vi "sv_Calculate Time and Angle Positions.vi"(0 "waveform in":waveform(dbl), 2 "reset?":bool, 5 "chirp settings":T1={"amplitude"=0.0, "frequency range"={"start (Hz)"=20.0, "stop (Hz)"=20000.0, "frequency spacing"=enum."Logarithmic"}, "sampling info"={"Fs"=50000.0, "chirp duration [s]"=3.0}, "initial states"={"frequency [Hz]"=20.0, "phase [rad]"=0.0, "elapsed time [s]"=0.0}, "frequency slope"=0.0, "maximum harmonic"=0, "prefix len [samples]"={"integer"=0, "fractional"=0.0}} {"frequency slope" format="%.2f"; "prefix len [samples]"."fractional" format="%.2p"; "initial states"."elapsed time [s]" format="%.2f"; "initial states"."phase [rad]" format="%.2f"; "initial states"."frequency [Hz]" format="%.2f"; "sampling info"."chirp duration [s]" format="%.2f"; "sampling info"."Fs" format="%.2p"; "frequency range"."stop (Hz)" format="%.2f"; "frequency range"."start (Hz)" format="%.2f"; "amplitude" format="%.2f"}, 11 "error in (no error)":errorcluster) -> (4 "waveform out":waveform(dbl), 6 "time array [s]":dbl[](array[numeric]), 8 "phase array [rad]":dbl[](array[numeric]), 10 "samples/rev":i32, 15 "error out":errorcluster)   [LabVIEW 2017, in "SoundVib_ContSweptSine.lvlib"]
uses:
  <vilib>/addons/Sound and Vibration/svt_Continuous Swept Sine/SoundVib_ContSweptSine.lvlib
  <vilib>/addons/_NISVFA/_Generation/subVIs/sv_Chirp Settings.ctl
  <vilib>/addons/Sound and Vibration/svt_Continuous Swept Sine/subVIs/sv_Continuous Swept-Sine Errors.ctl
  <vilib>/addons/_NISVFA/_Generation/SoundVib_Generation.lvlib
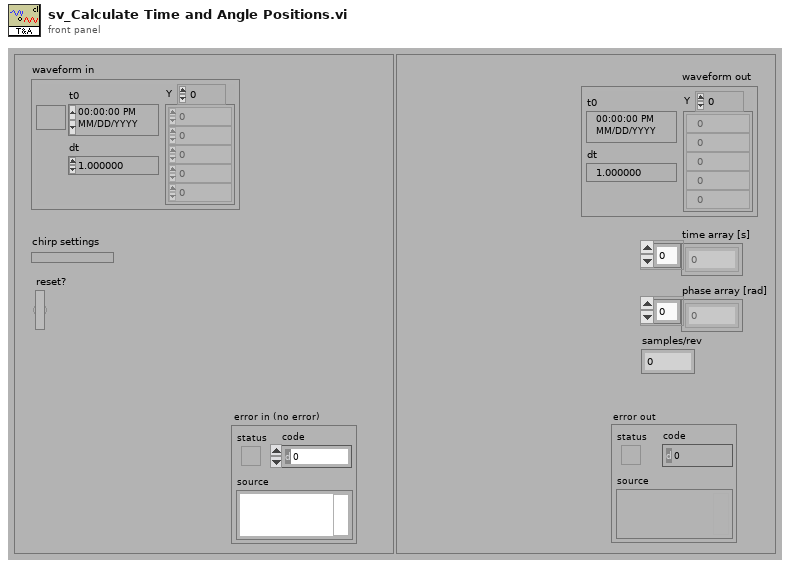
[diagram p1: front panel]
types:
  T1 = typedef "SoundVib_Generation.lvlib/sv_Chirp Settings.ctl" = cluster{"amplitude":dbl, "frequency range":cluster{"start (Hz)":dbl, "stop (Hz)":dbl, "frequency spacing":enum16{"Linear", "Logarithmic"}}, "sampling info":cluster{"Fs":dbl, "chirp duration [s]":dbl}, "initial states":cluster{"frequency [Hz]":dbl, "phase [rad]":dbl, "elapsed time [s]":dbl}, "frequency slope":dbl, "maximum harmonic":i32, "prefix len [samples]":cluster{"integer":u32, "fractional":dbl}}
  T2 = typedef "SoundVib_ContSweptSine.lvlib/sv_Continuous Swept-Sine Errors.ctl" = enum16{"Invalid AI sampling rate", "Item not found", "Invalid initial phase"}
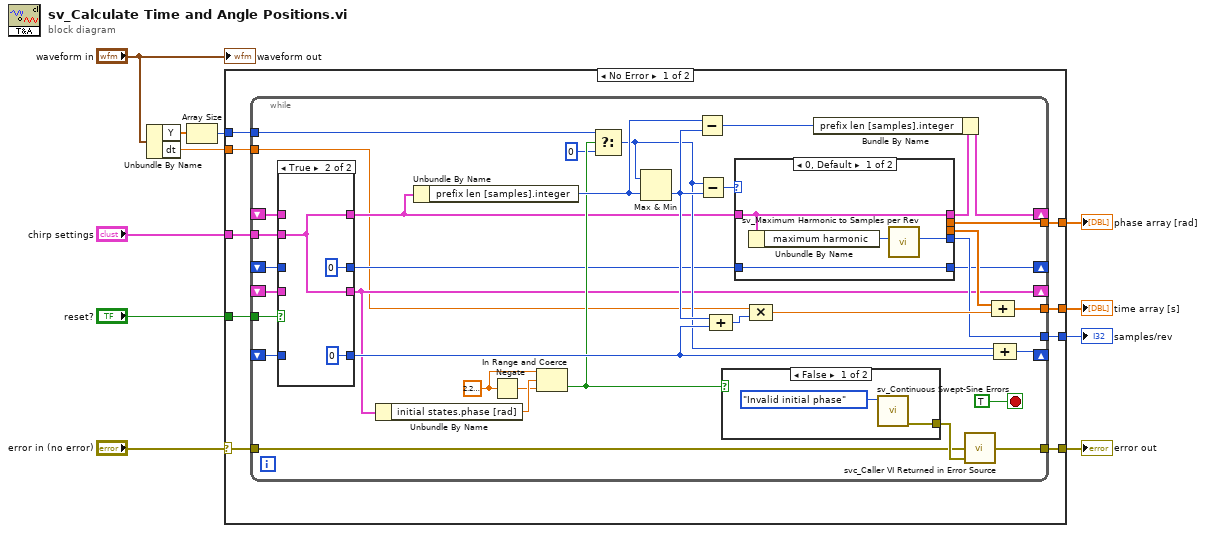
[diagram p0: block diagram]
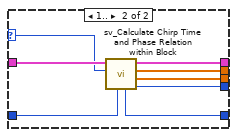
[diagram p3: hidden frame]
diagram:
  n1 = Unbundle By Name("waveform in") -> ("Y"=w4:dbl[], "dt"=w1:dbl)
  n2 = Array Size(array=w4) -> (size(s)=w2:i32)
  n3 = case shown="No Error" "error in (no error)" {
    selector: "error in (no error)" -> [w15 w78]
    tunnel: [w14 w78] -> w10
    tunnel: "chirp settings" -> [w19 _]
    tunnel: "reset?" -> [w20 _]
    tunnel: [w18 _] -> w8
    tunnel: [w17 _] -> w7
    tunnel: [w16 _] -> w6
    tunnel: w2 -> [w13 _]
    tunnel: w1 -> [w12 _]
    frame No Error {
      n4 = while {
        tunnel: w20 -> [w55]
        tunnel: w19 -> [w28]
        shift-right: [w41] -> _
        shift-left: _ -> [w54]
        shift-right: [w51] -> _
        shift-left: _ -> [w52]
        tunnel: [w45] -> w18
        tunnel: [w44] -> w17
        tunnel: [w40] -> w16
        tunnel: w15 -> [w34]
        tunnel: [w33] -> w14
        shift-right: [w26] -> _
        shift-left: _ -> [w27]
        shift-right: [w25] -> _
        shift-left: _ -> [w24]
        tunnel: w13 -> [w22]
        tunnel: w12 -> [w21]
        stop <- TRUE stop-if-true
        w36 = 2.220446049250313e-16
        n5 = case shown="True" w55 {
          tunnel: w28 -> [_ w76]
          tunnel: [w74 w76] -> w29
          tunnel: w54 -> [w74 _]
          tunnel: [w73 0] -> w49
          tunnel: w52 -> [w73 _]
          tunnel: [w72 w76] -> w26
          tunnel: w27 -> [w72 _]
          tunnel: [w71 0 ("# of even-angle samples out")] -> w23
          tunnel: w24 -> [w71 _]
          frame False {
          }
          frame True {
          }
        }
        n6 = Unbundle By Name(w26) -> ("initial states.phase [rad]"=w38:dbl)
        n7 = Unbundle By Name(w29) -> ("prefix len [samples].integer"=w39:u32)
        n8 = Negate(x=w36) -> (-x=w37:dbl)
        n9 = In Range and Coerce(upper limit=w36, x=w38, lower limit=w37) -> (In Range?=w32:bool)  [unwired: 1 out]
        n10 = Select(t=w22, s=w32, f=0) -> (s? t:f=w31:i32)
        n11 = Max & Min(x=w31, y=w39) -> (min(x,y)=w50:u32)  [unwired: 1 out]
        n12 = Subtract(x=w39, y=w50) -> (x-y=w42:u32)
        n13 = Subtract(x=w31, y=w50) -> (x-y=w53:u32)
        n14 = Compound Arithmetic op=ADD(w50, w49) -> (w48:u32)
        n15 = case shown="False" w32 {
          tunnel: [w57 _] -> w35
          frame False {
            n16 = call <vilib>:"sv_Continuous Swept-Sine Errors.vi"("continuous swept-sine error"=sv_Continuous_Swept-Sine_Errors."Invalid initial phase") -> ("error out"=w57:errorcluster)  [unwired: 10 in]
          }
          frame True {
          }
        }
        n17 = case shown="0, Default" w53 {
          selector: w53 -> [_ w68]
          tunnel: w29 -> [w62 w70]
          tunnel: [w62 w69] -> w43
          tunnel: [_ w67] -> w45
          tunnel: [_ w66] -> w47
          tunnel: [w60 w65] -> w40
          tunnel: [w59 w64] -> w25
          tunnel: w23 -> [w59 w63]
          frame 0, Default {
            n18 = Unbundle By Name(w62) -> ("maximum harmonic"=w61:i32)
            n19 = call <vilib>:"sv_Maximum Harmonic to Samples per Rev.vi"("maximum harmonic"=w61) -> ("samples/rev"=w60:i32)  [unwired: 10 in]
          }
          frame 1.. {
            n20 = call <vilib>:"sv_Calculate Chirp Time and Phase Relation within Block.vi"("# of even-angle samples in"=w63, "block size [samples]"=w68, "continuous swept-sine settings"=w70) -> ("samples/rev"=w65:i32, "time instances [s]"=w66:dbl[], "phases [rad]"=w67:dbl[], "continuous swept-sine settings out"=w69:T1, "# of even-angle samples out"=w64:i32)  [unwired: 4 in]
          }
        }
        n21 = Compound Arithmetic op=MULTIPLY(w21, w48) -> (w46:dbl)
        n22 = Bundle By Name(cluster=w43, "prefix len [samples].integer"=w42) -> (w41:T1)
        n23 = call <vilib>:"svc_Caller VI Returned in Error Source.vi"("warning input to caller"=w35, "error in (no error)"=w34) -> ("error out"=w33:errorcluster)  [unwired: 3 in]
        n24 = Compound Arithmetic op=ADD(w47, w46) -> (w44:dbl[])
        n25 = Compound Arithmetic op=ADD(w31, w49) -> (w51:i32)
      }
    }
    frame Error {
    }
  }
  "error out" <- w10
  "phase array [rad]" <- w8
  "time array [s]" <- w7
  "samples/rev" <- w6
  "waveform out" <- "waveform in"
